vi "startStanDt.vi"(8 "error in (no error)":errorcluster, 10 "duration":dbl, 11 "ElectrometerController in":refnum<class "ElectrometerController.lvclass">) -> (0 "error out":errorcluster, 3 "ElectrometerController out":refnum<class "ElectrometerController.lvclass">)   [LabVIEW 2016, in "ElectrometerController.lvclass"]
uses:
  ElectrometerController.lvclass
  Electrometer/State/ElectrometerState.lvclass
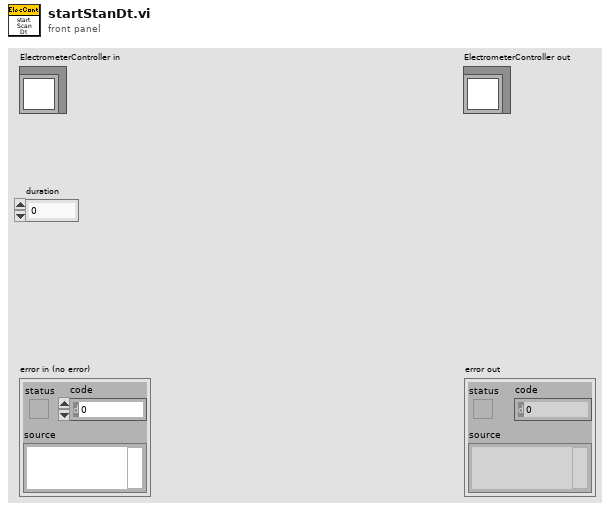
[diagram p1: front panel]
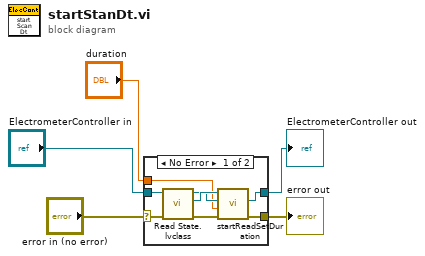
[diagram p0: block diagram]
diagram:
  n1 = case shown="No Error" "error in (no error)" {
    selector: "error in (no error)" -> [w6 w15]
    tunnel: [w10 w15] -> w4
    tunnel: [w9 w14] -> w2
    tunnel: "ElectrometerController in" -> [w7 w14]
    tunnel: "duration" -> [w11 _]
    frame No Error {
      n2 = call-dynamic "Read State.lvclass.vi"("error in (no error)"=w6, "ElectrometerController in"=w7) -> ("error out"=w8:errorcluster, "ElectrometerState"=w13:refnum<class "ElectrometerState.lvclass">, "ElectrometerController out"=w12:refnum<class "ElectrometerController.lvclass">)  [unwired: 7 in]
      n3 = call-dynamic "startReadSetDuration.vi"("error in (no error)"=w8, "duration"=w11, "ElectrometerController in"=w12, "State in"=w13) -> ("error out"=w10:errorcluster, "ElectrometerController. out"=w9:refnum<class "ElectrometerController.lvclass">)  [unwired: 5 in, 1 out]
    }
    frame Error {
    }
  }
  "error out" <- w4
  "ElectrometerController out" <- w2
